vi "Graph_2_Signal.vi"(9 "y":timestamp, 10 "Dynamic Data 2":dbl, 11 "Dynamic Data 1":dbl) -> (3 "Signals":dynamicdata(graph))   [LabVIEW 2019]
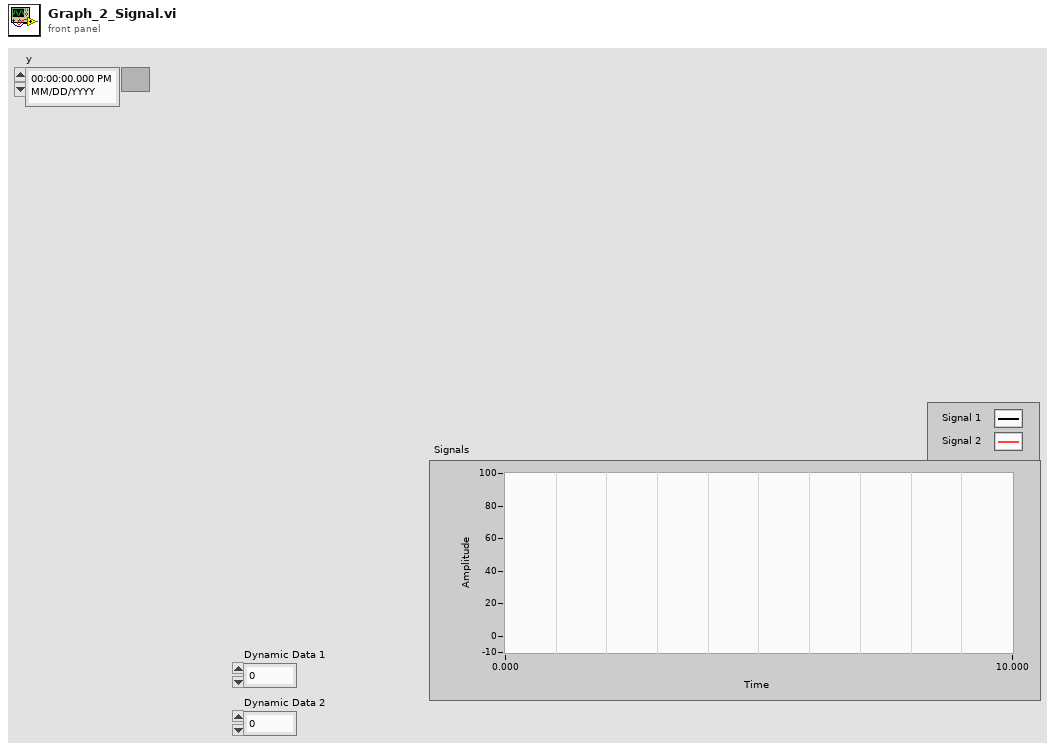
[diagram p1: front panel]
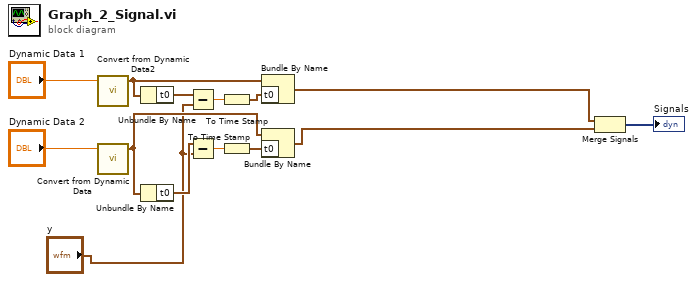
[diagram p0: block diagram]
diagram:
  n1 = call "Convert from Dynamic Data2"("Dynamic Data Type"="Dynamic Data 1") -> ("Waveform"=w10:waveform(dbl))  [unwired: 3 in]
  n2 = call "Convert from Dynamic Data"("Dynamic Data Type"="Dynamic Data 2") -> ("Waveform"=w14:waveform(dbl))  [unwired: 3 in]
  n3 = Unbundle By Name ("Get Waveform Components 2")(w10) -> ("t0"=w7:timestamp)
  n4 = Unbundle By Name ("Get Waveform Components")(w14) -> ("t0"=w11:timestamp)
  n5 = Subtract ("Subtract 2")(x=w7, y="y") -> (x-y=w9:dbl)
  n6 = Subtract(x=w11, y="y") -> (x-y=w13:dbl)
  n7 = To Time Stamp ("To Time Stamp 2")(1:w9) -> (0:w8:timestamp)
  n8 = To Time Stamp(1:w13) -> (0:w12:timestamp)
  n9 = Bundle By Name ("Build Waveform 2")(cluster=w10, "t0"=w8) -> (w3:waveform(dbl))
  n10 = Bundle By Name ("Build Waveform")(cluster=w14, "t0"=w12) -> (w2:waveform(dbl))
  n11 = Merge Signals(w3, w2) -> (→"Signals":dynamicdata)
